vi "Completion Score.vi"(11 "Symbols":T1[](array[typedef])) -> (3 "Score":u64)   [LabVIEW 2020]
uses:
  Open Symbol.ctl
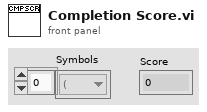
[diagram p1: front panel]
types:
  T1 = typedef "Open Symbol.ctl" = enum16{"(", "[", "{", "<"}
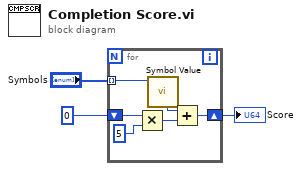
[diagram p0: block diagram]
diagram:
  n1 = for {
    tunnel: "Symbols" -> [w7] mode=indexing
    shift-right: [w4] -> w1
    shift-left: u64 0 -> [w9]
    n2 = Multiply(x=w9, y=u64 5) -> (x*y=w6:u64)
    n3 = call "Symbol Value.vi"("Open Symbol"=w7) -> ("Incomplete Val"=w5:u64)  [unwired: 9 in, 1 out]
    n4 = Add(x=w5, y=w6) -> (x+y=w4:u64)
  }
  "Score" <- w1
